vi "Rose_Analysis_03.vi"() -> (5 "Plug in titles":string[](array[string]), 7 "Plug in values":string[](array[string]))   [LabVIEW 2010]
uses:
  Globals/Meas_global.vi
  Globals/LDA_meas_global_1.vi
  Globals/Plug_in_data_global.vi
panel:
  out "Correlation:(tweaked):(ppm^2)":string
  out "Samples Slipped":i32
  in  "No of samples:Averaged:Together:":i32=5
  out "Slip (ms)":dbl format="%.2f"
  # "The slip value is set  at the measurement input panel"
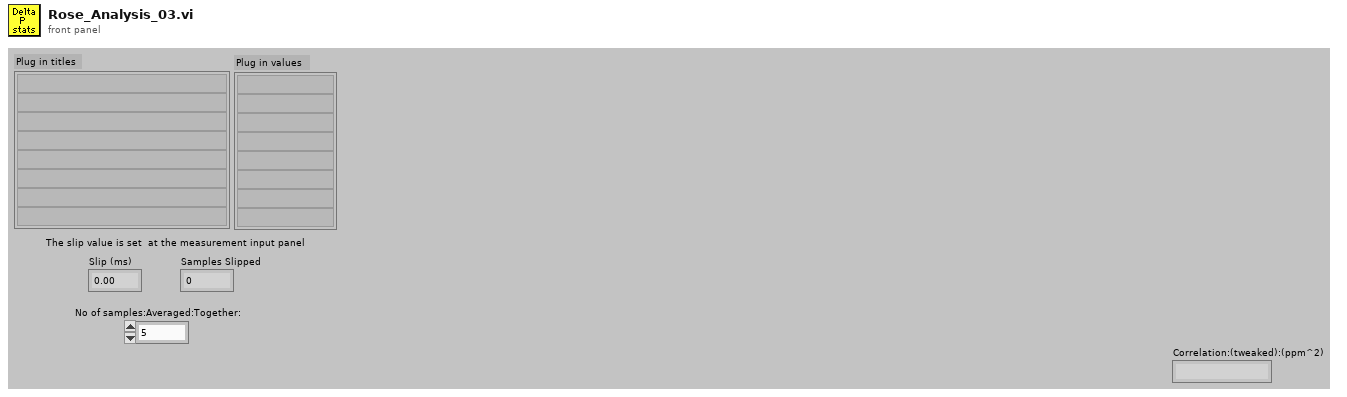
[diagram p1: front panel]
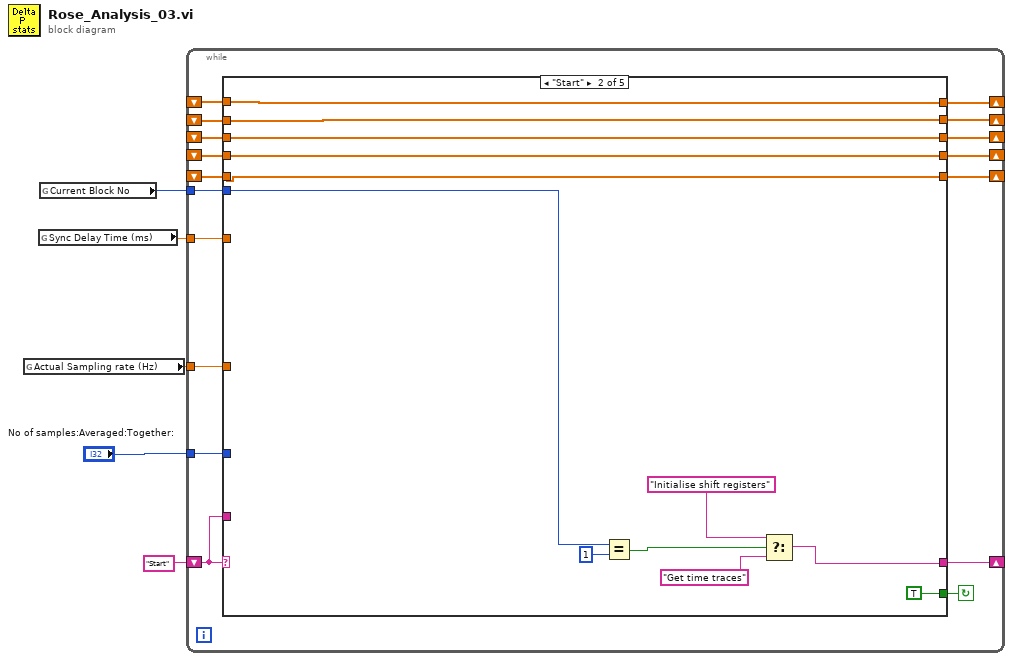
[diagram p0: block diagram]
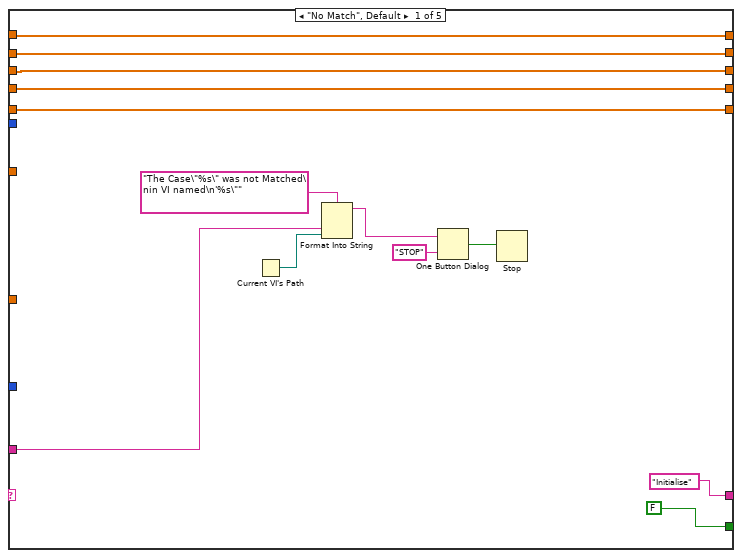
[diagram p2: hidden frame]
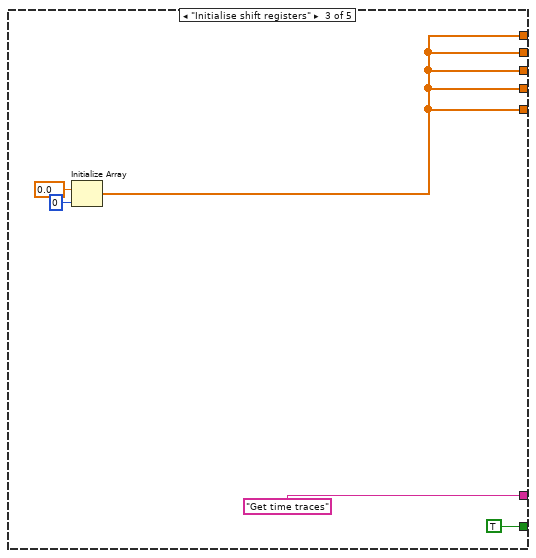
[diagram p3: hidden frame]
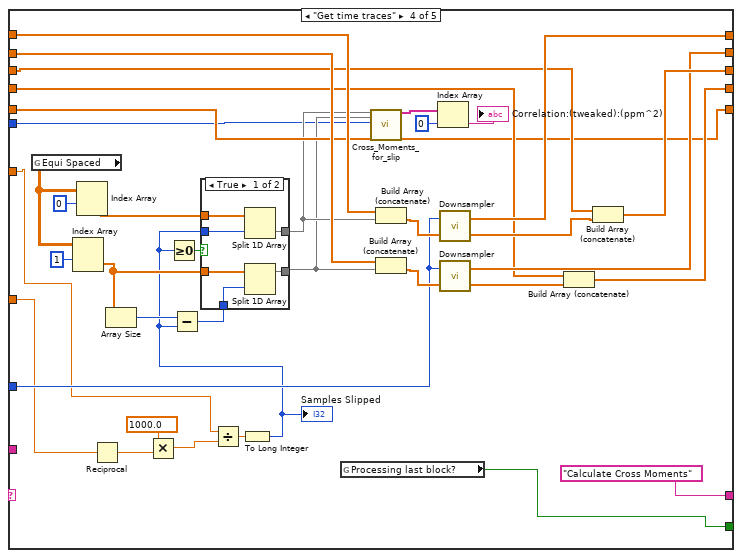
[diagram p4: hidden frame]
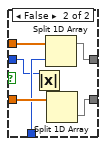
[diagram p5: hidden frame]
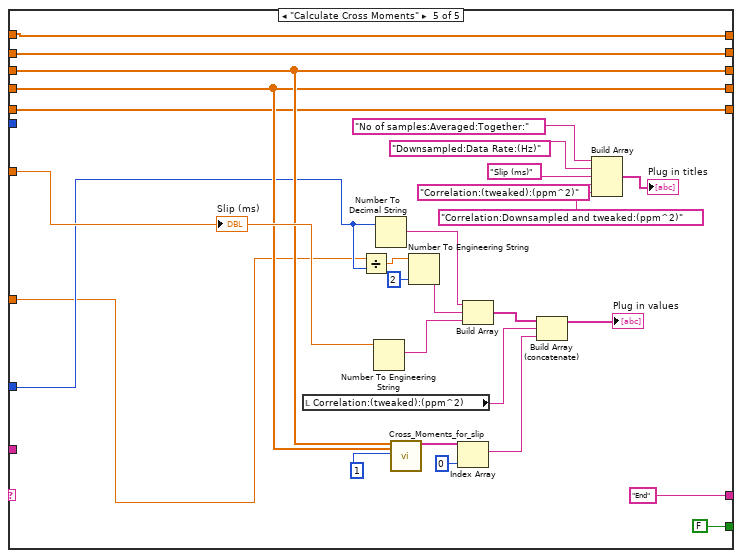
[diagram p6: hidden frame]
diagram:
  n1 = global read "Meas_global.vi" "Actual Sampling rate (Hz)"() -> (w2:dbl)
  n2 = global read "LDA_meas_global_1.vi" "Sync Delay Time (ms)"() -> (w3:dbl)
  n3 = global read "Meas_global.vi" "Current Block No"() -> (w1:i32)
  n4 = while {
    shift-left: "Start" -> [w20]
    shift-right: [w21] -> _
    shift-right: [w18] -> _
    shift-left: _ -> [w19]
    shift-right: [w17] -> _
    shift-left: _ -> [w16]
    shift-right: [w14] -> _
    shift-left: _ -> [w15]
    shift-right: [w13] -> _
    shift-left: _ -> [w12]
    tunnel: "No of samples:Averaged:Together:" -> [w11]
    tunnel: w2 -> [w10]
    tunnel: w3 -> [w9]
    shift-right: [w7] -> _
    shift-left: _ -> [w8]
    tunnel: w1 -> [w6]
    stop <- w22 continue-if-true
    n5 = case shown="\"Start\"" w20 {
      tunnel: [FALSE TRUE TRUE w68 FALSE] -> w22
      tunnel: ["Initialise" w39 "Get time traces" ("f") "Calculate Cross Moments" "End"] -> w21
      tunnel: w20 -> [w30 _ _ _ _]
      tunnel: w19 -> [w27 w47 _ w82 w122]
      tunnel: [w27 w47 w48 w80 w122] -> w18
      tunnel: [w26 w46 w48 w74 w121] -> w17
      tunnel: w16 -> [w26 w46 _ w78 w121]
      tunnel: w15 -> [w25 w45 _ w76 w120]
      tunnel: [w25 w45 w48 w75 w120] -> w14
      tunnel: [w24 w44 w48 w71 w119] -> w13
      tunnel: w12 -> [w24 w44 _ w72 w119]
      tunnel: w11 -> [_ _ _ w69 w117]
      tunnel: w10 -> [_ _ _ w62 w110]
      tunnel: w9 -> [_ _ _ w65 w123]
      tunnel: w8 -> [w23 w36 _ w60 w109]
      tunnel: [w23 w36 w48 w59 w109] -> w7
      tunnel: w6 -> [_ w37 _ w56 _]
      frame "No Match", Default {
        n6 = Current VI's Path() -> (path=w29:path)
        n7 = Format Into String(format string="The Case\"%s\" was not Matched\nin VI named\n'%s\"" ("Format String"), w30, w29) -> (resulting string=w33:string)  [unwired: 2 in, 1 out]
        n8 = One Button Dialog(message=w33, button name ("OK")="STOP") -> (true=w31:bool)
        n9 = Stop(stop? (T)=w31) -> ()
      }
      frame "Start" {
        n10 = Equal?(x=w37, y=1) -> (x = y?=w42:bool)
        n11 = Select(t="Initialise shift registers", s=w42, f="Get time traces") -> (s? t:f=w39:string)
      }
      frame "Initialise shift registers" {
        n12 = Initialize Array(0.0 ("element"), 0 ("dimension size")) -> (w48:dbl[])
      }
      frame "Get time traces" {
        n13 = global read "Plug_in_data_global.vi" "Equi Spaced"() -> (w70:dbl[][])
        n14 = Index Array(array=w70, index (row)=1) -> (element=w86:dbl[])  [unwired: 1 in]
        n15 = Index Array(array=w70, index (row)=0) -> (element=w87:dbl[])  [unwired: 1 in]
        n16 = Reciprocal(x=w62) -> (1/x=w61:dbl)
        n17 = Array Size(array=w86) -> (size(s)=w85:i32)
        n18 = Multiply(x=1000.0, y=w61) -> (x*y=w66:dbl)
        n19 = Divide(x=w65, y=w66) -> (x/y=w64:dbl)
        n20 = To Long Integer(number=w64) -> (32bit integer=w63:i32)
        "Samples Slipped" <- w63
        n21 = Greater Or Equal To 0?(x=w63) -> (x >= 0?=w83:bool)
        n22 = Subtract(x=w85, y=w63) -> (x-y=w84:i32)
        n23 = case shown="True" w83 {
          tunnel: w87 -> [w96 w103]
          tunnel: w86 -> [w95 w102]
          tunnel: w84 -> [w94 w101]
          tunnel: w63 -> [w93 w100]
          tunnel: [w92 w99] -> w58
          tunnel: [w91 w98] -> w57
          frame True {
            n24 = Split 1D Array(array=w96, index=w93) -> (second subarray=w92:dbl[])  [unwired: 1 out]
            n25 = Split 1D Array(array=w95, index=w94) -> (first subarray=w91:dbl[])  [unwired: 1 out]
          }
          frame False {
            n26 = Absolute Value(x=w100) -> (abs(x)=w97:i32)
            n27 = Split 1D Array(array=w103, index=w101) -> (first subarray=w99:dbl[])  [unwired: 1 out]
            n28 = Split 1D Array(array=w102, index=w97) -> (second subarray=w98:dbl[])  [unwired: 1 out]
          }
        }
        n29 = global read "Meas_global.vi" "Processing last block?"() -> (w68:bool)
        n30 = call "Cross_Moments_for_slip.vi"("U"=w58, "W"=w57, "Block No"=w56, "Shift in"=w60) -> ("Correlations Only"=w54:string[], "Shift out"=w59:dbl[])  [unwired: 14 out]
        n31 = Build Array (concatenate)(w82, w58) -> (w81:dbl[])
        n32 = Build Array (concatenate)(w78, w57) -> (w79:dbl[])
        n33 = Index Array(array=w54, index=0) -> (element=→"Correlation:(tweaked):(ppm^2)":string)
        n34 = call "Downsampler.vi"("Input Array"=w81, "Averaging samples"=w69) -> ("Downsampled Array"=w77:dbl[], "Samples remaining"=w80:dbl[])
        n35 = call "Downsampler.vi"("Input Array"=w79, "Averaging samples"=w69) -> ("Downsampled Array"=w73:dbl[], "Samples remaining"=w74:dbl[])
        n36 = Build Array (concatenate)(w72, w73) -> (w71:dbl[])
        n37 = Build Array (concatenate)(w76, w77) -> (w75:dbl[])
      }
      frame "Calculate Cross Moments" {
        n38 = local read "Correlation:(tweaked):(ppm^2)"() -> (w104:string)
        n39 = Divide(x=w110, y=w117) -> (x/y=w116:dbl)
        n40 = Number To Engineering String(4:w123) -> (0:w111:string)  [unwired: 3 out]
        n41 = Number To Decimal String(number=w117) -> (decimal integer string=w114:string)  [unwired: 1 out]
        n42 = call "Cross_Moments_for_slip.vi"("U"=w120, "W"=w119, "Block No"=1) -> ("Correlations Only"=w107:string[])  [unwired: 1 in, 15 out]
        n43 = Number To Engineering String(2:i16 2 ("precision (6)"), 4:w116) -> (0:w113:string)  [unwired: 2 out]
        n44 = Index Array(array=w107, index=0) -> (element=w105:string)
        n45 = Build Array(w114, w113, w111) -> (w124:string[])
        n46 = Build Array (concatenate)(w124, w104, w105) -> (→"Plug in values":string[])
        n47 = Build Array("No of samples:Averaged:Together:" ("element"), "Downsampled:Data Rate:(Hz)" ("element"), "Slip (ms)" ("element"), "Correlation:(tweaked):(ppm^2)", "Correlation:Downsampled and tweaked:(ppm^2)") -> (→"Plug in titles":string[])
        "Slip (ms)" <- w123
      }
    }
  }
